vi "splitter for cDAQ Input.vi"(11 "VALUE":dbl[](array[numeric])) -> (1 "MOD 3":dbl[](array[numeric]), 2 "MOD 2":dbl[](array[numeric]), 3 "MOD 1":dbl[](array[numeric]))   [LabVIEW 2019]
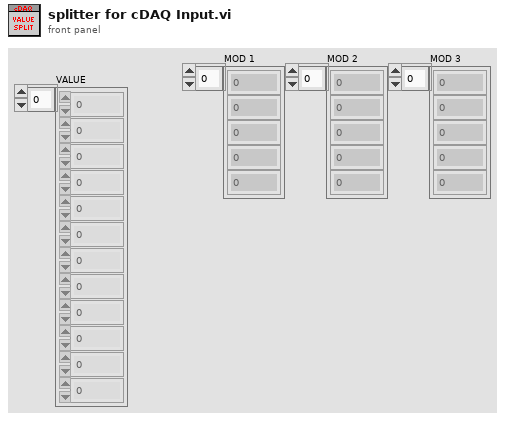
[diagram p1: front panel]
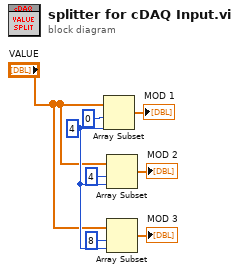
[diagram p0: block diagram]
diagram:
  w6 = 4 ("length")
  n1 = Array Subset(array="VALUE", index=0, length=w6) -> (→"MOD 1":dbl[])
  n2 = Array Subset(array="VALUE", index=4, length=w6) -> (→"MOD 2":dbl[])
  n3 = Array Subset(array="VALUE", index=8, length=w6) -> (→"MOD 3":dbl[])
